vi "Hide Unused.vi"(7 "Hide unused":bool, 12 "DIO ref":refnum<vi>) -> (14 "DIO ref out":refnum<vi>)   [LabVIEW 2015, in "Digital I-O.xctl"]
uses:
  Digital I-O.xctl
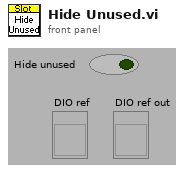
[diagram p1: front panel]
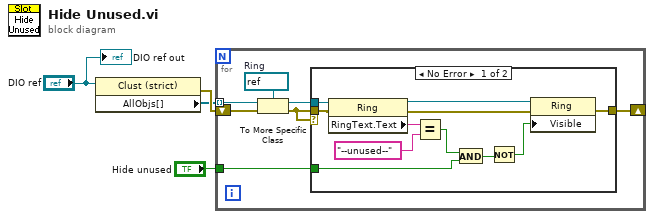
[diagram p0: block diagram]
diagram:
  n1 = property class="Clust (strict)"(reference="DIO ref") -> (error out=w3:errorcluster, "AllObjs[]"=w2:refnum<vi>[])  [unwired: 1 in, 1 out]
  n2 = for {
    tunnel: w2 -> [w6] mode=indexing
    tunnel: "Hide unused" -> [w10]
    shift-right: [w9] -> _
    shift-left: w3 -> [w7]
    w11 = refnum<vi> refnum  # Ring
    n3 = To More Specific Class(target class=w11, reference=w6, error in=w7) -> (specific class reference=w5:refnum<vi>, error out=w8:errorcluster)
    n4 = case shown="No Error" w8 {
      tunnel: w5 -> [w22 _]
      tunnel: w10 -> [w18 _]
      tunnel: w8 -> [w16 _]
      tunnel: [w14 _] -> w9
      frame No Error {
        n5 = property class="Ring"(reference=w22, error in=w16) -> (reference out=w19:refnum<vi>, error out=w15:errorcluster, "RingText.Text"=w21:string)
        n6 = Equal?(x=w21, y="--unused--") -> (x = y?=w13:bool)
        n7 = And(x=w13, y=w18) -> (x .and. y?=w17:bool)
        n8 = Not(x=w17) -> (.not. x?=w12:bool)
        n9 = property class="Ring"(reference=w19, error in=w15, "Visible"=w12) -> (error out=w14:errorcluster)  [unwired: 1 out]
      }
      frame Error {
      }
    }
  }
  "DIO ref out" <- "DIO ref"
